vi "UpdateRequestTime.vi"(7 "TimeType":enum16{"StartTime", "AckTime", "FulfilledTime"}(ring), 8 "error in":errorcluster, 9 "Time":timestamp, 10 "RequestID":string) -> (0 "error out":errorcluster)   [LabVIEW 2015, in "DatabaseApi.lvlib"]
uses:
  DatabaseApi.lvlib
  TypeDef/Request/RequestsTableColumnNamesRing.ctl
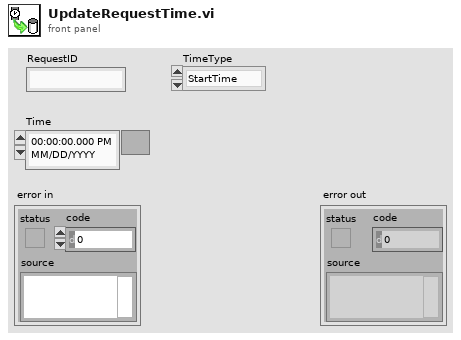
[diagram p1: front panel]
types:
  T1 = typedef "DatabaseApi.lvlib/RequestsTableColumnNamesRing.ctl" = enum16{"RequestID", "PersonnelType", "StartTime", "StartName", "AckTime", "AckName", "FulfilledTime", "FulfilledName", "Description", "Room Number", "Request Type", "Alarm"}
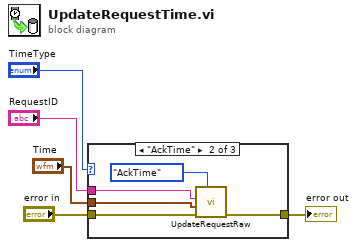
[diagram p0: block diagram]
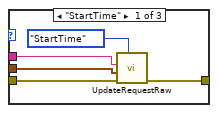
[diagram p2: hidden frame]
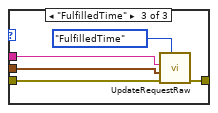
[diagram p3: hidden frame]
diagram:
  n1 = case shown="\"AckTime\"" "TimeType" {
    tunnel: "error in" -> [w10 w15 w20]
    tunnel: "RequestID" -> [w9 w14 w19]
    tunnel: [w8 w13 w18] -> w3
    tunnel: "Time" -> [w6 w11 w16]
    frame "StartTime" {
      n2 = call "UpdateRequestRaw.vi"("Data to update"=RequestsTableColumnNamesRing."StartTime", "error in"=w10, "data"=w6, "RequestID"=w9) -> ("error out"=w8:errorcluster)  [unwired: 7 in]
    }
    frame "AckTime" {
      n3 = call "UpdateRequestRaw.vi"("Data to update"=RequestsTableColumnNamesRing."AckTime", "error in"=w15, "data"=w11, "RequestID"=w14) -> ("error out"=w13:errorcluster)  [unwired: 7 in]
    }
    frame "FulfilledTime" {
      n4 = call "UpdateRequestRaw.vi"("Data to update"=RequestsTableColumnNamesRing."FulfilledTime", "error in"=w20, "data"=w16, "RequestID"=w19) -> ("error out"=w18:errorcluster)  [unwired: 7 in]
    }
  }
  "error out" <- w3
